vi "BonOMM-SAOMM.Test.vi"() -> ()   [LabVIEW 2011] (continued)
            stop <- w2768 stop-if-true
            # "Commandes Externes sur le PORT SÉRIE et TCP/IP"
            n5059 = local read "CmdFIFO"() -> (w2769:T14)
            n5060 = Array Size(array=w2769) -> (size(s)=w2771:i32)
            n5061 = Greater Than 0?(x=w2771) -> (x > 0?=w2770:bool)
            n5062 = case shown="True" w2770 {
              tunnel: w2769 -> [_ w2779]
              frame False {
                n5063 = local write "ActiveCmd"(T15 {"CmdAct"="", "CmdArgs"="", "Source"=""} ("ActiveCmd")) -> ()
                "CmdPending" <- FALSE
              }
              frame True {
                w2775 = u32 0 ("Output Code")
                # "Enlève les erreurs ..."
                # "Enlève l'élément du FIFO"
                n5064 = stacked-sequence {
                  tunnel: w2779 -> [_ w2793 _]
                  tunnel: [_ w2788 _] -> w2778
                  tunnel: [_ w2787 _] -> w2777
                  tunnel: [_ w2786 _] -> w2776
                  frame #0 {
                    n5065 = control-ref of="FIFO actif"() -> (w2780:refnum<vi>)
                    n5066 = call "Fifo-Wait4Flag.vi"("Raise Flag ?"=TRUE, "Ctl Refnum IN"=w2780) -> ()  [unwired: 8 in, 2 out]
                  }
                  frame #1 {
                    n5067 = local read "CmdDone"() -> (w2784:T14)
                    n5068 = Delete From Array(array=w2793, length=1, index=0) -> (deleted portion=w2789:T14, array with subset deleted=w2790:T14)
                    n5069 = local write "CmdFIFO"(w2790) -> ()
                    n5070 = Index Array(array=w2789) -> (element=w2785:T15)  [unwired: 1 in]
                    "ActiveCmd" <- w2785
                    n5071 = call "PCE-Archive.vi"("Nouvelle Commande"=w2785, "MaxLength"=3, "CmdDone IN"=w2784) -> ("CmdDone OUT"=w2783:T14)  [unwired: 8 in]
                    n5072 = Unbundle By Name(w2785) -> ("CmdAct"=w2788:string, "CmdArgs"=w2787:string, "Source"=w2786:string)
                    n5073 = local write "CmdDone"(w2783) -> ()
                  }
                  frame #2 {
                    n5074 = local write "FIFO actif"(FALSE) -> ()
                  }
                }
                n5075 = stacked-sequence {
                  tunnel: w2778 -> [w2797 _]
                  tunnel: w2777 -> [w2796 _]
                  tunnel: w2776 -> [w2795 w3138]
                  frame #0 {
                    # "Effectue la commande ..."
                    n5076 = case shown="\"EFOY \"" w2797 {
                      tunnel: w2796 -> [_ w2803 w2899 w2907 w2945 w3049 w3057 _]
                      tunnel: w2795 -> [_ _ _ _ _ _ _ _]
                      frame Default {
                        n5077 = local write "ANSW"("Commande non reconnue" ("ANSW")) -> ()
                      }
                      frame "ETCS" {
                        # "Commandes vers TCS"
                        n5078 = call "ETCS_decodeur.vi"("chaine entree"=w2803) -> ("Args"=w2800:dbl[], "nb args"=w2804:i32)  [unwired: 1 out]
                        n5079 = Delete From Array(array=w2800, index=0 ("indice")) -> (deleted portion=w2801:dbl, array with subset deleted=w2799:dbl[])  [unwired: 1 in]
                        n5080 = To Long Integer(number=w2801) -> (32bit integer=w2805:i32)
                        n5081 = case shown="27" w2805 {
                          selector: w2805 -> [_ w2816 _ w2881]
                          tunnel: w2804 -> [_ w2817 w2851 _]
                          tunnel: w2799 -> [_ w2815 _ w2880]
                          frame 0, Default {
                            w2806 = u32 128 ("Bit to add")
                            n5082 = local read "Warning Code"() -> (w2810:u32)
                            n5083 = local read "FIFO d'erreur"() -> (w2808:T7)
                            n5084 = local read "Error Code"() -> (w2809:u32)
                            n5085 = call "Error_Format.vi"("FIFO IN"=w2808, "Error Code IN"=w2809, "Warning Code IN"=w2810, "Error Bit"=w2806, "Warning Bit"=w2806, "Source"="ETCS", "Comment"="Commande non-supportée/indéfinie") -> ("FIFO OUT"=w2811:T7, "Error Code OUT"=w2812:u32, "Warning Code OUT"=w2813:u32)  [unwired: 10 in]
                            n5086 = local write "Warning Code"(w2813) -> ()
                            n5087 = local write "FIFO d'erreur"(w2811) -> ()
                            n5088 = local write "Error Code"(w2812) -> ()
                          }
                          frame 6, 14..16, 22 {
                            # "Vérifie le nombre d'arguments ..."
                            # "Envoir des commandes sans gestions ni réponse de TCS"
                            n5089 = case shown="6" w2816 {
                              tunnel: w2817 -> [w2843 w2844 w2849]
                              tunnel: [w2841 w2845 w2847] -> w2818
                              frame Default {
                                n5090 = Equal?(x=w2843, y=1) -> (x = y?=w2841:bool)
                              }
                              frame 6 {
                                n5091 = Equal?(x=w2844, y=3) -> (x = y?=w2845:bool)
                              }
                              frame 14 {
                                n5092 = Equal?(x=w2849, y=4) -> (x = y?=w2847:bool)
                              }
                            }
                            n5093 = case shown="True" w2818 {
                              tunnel: w2815 -> [_ w2826]
                              tunnel: w2816 -> [_ w2825]
                              frame False {
                                # "Nombre d'arguments incorrect"
                                n5094 = local read "Error Code"() -> (w2821:u32)
                                n5095 = Or(x=w2821, y=u32 128) -> (x .or. y?=w2820:u32)
                                n5096 = local write "Error Code"(w2820) -> ()
                              }
                              frame True {
                                n5097 = local read "TCS VRN"() -> (w2824:refnum<visa-resource-name>)
                                n5098 = control-ref of="TCS actif"() -> (w2822:refnum<vi>)
                                n5099 = call "EXCOM-CMD.vi"("VRN IN"=w2824, "Bool Refnum"=w2822, "Commande #"=w2825, "Args"=w2826) -> ("VRN OUT"=w2823:refnum<visa-resource-name>, "Error OUT"=w2827:errorcluster)  [unwired: 9 in, 1 out]
                                n5100 = local write "TCS VRN"(w2823) -> ()
                                n5101 = case shown="Error" w2827 {
                                tunnel: w2825 -> [_ w2838]
                                frame No Error {
                                }
                                frame Error {
                                w2828 = u32 4
                                n5102 = local read "Warning Code"() -> (w2834:u32)
                                n5103 = local read "FIFO d'erreur"() -> (w2836:T7)
                                n5104 = local read "Error Code"() -> (w2835:u32)
                                n5105 = Number To Decimal String(number=w2838) -> (decimal integer string=w2837:string)  [unwired: 1 in]
                                n5106 = Concatenate Strings("Erreur lors de l'envoie de la commande #", w2837, ", vérifiez la communication sur le port TCS C ...") -> (w2833:string)
                                n5107 = call "Error_Format.vi"("FIFO IN"=w2836, "Error Code IN"=w2835, "Warning Code IN"=w2834, "Error Bit"=w2828, "Warning Bit"=w2828, "Source"="ETCS", "Comment"=w2833) -> ("FIFO OUT"=w2832:T7, "Error Code OUT"=w2831:u32, "Warning Code OUT"=w2830:u32)  [unwired: 10 in]
                                n5108 = local write "Warning Code"(w2830) -> ()
                                n5109 = local write "FIFO d'erreur"(w2832) -> ()
                                n5110 = local write "Error Code"(w2831) -> ()
                                }
                                }
                              }
                            }
                          }
                          frame 4 {
                            # "Commande de rotation semie-automatisée ..."
                            n5111 = Equal?(x=w2851, y=2) -> (x = y?=w2852:bool)
                            n5112 = case shown="True" w2852 {
                              frame False {
                                n5113 = local read "Warning Code"() -> (w2859:u32)
                                n5114 = local read "FIFO d'erreur"() -> (w2861:T7)
                                n5115 = local read "Error Code"() -> (w2860:u32)
                                n5116 = call "Error_Format.vi"("FIFO IN"=w2861, "Error Code IN"=w2860, "Warning Code IN"=w2859, "Warning Bit"=u32 128, "Source"="ETCS", "Comment"="Nombre d'arguments incompatibles") -> ("FIFO OUT"=w2857:T7, "Error Code OUT"=w2856:u32, "Warning Code OUT"=w2855:u32)  [unwired: 11 in]
                                n5117 = local write "Warning Code"(w2855) -> ()
                                n5118 = local write "FIFO d'erreur"(w2857) -> ()
                                n5119 = local write "Error Code"(w2856) -> ()
                              }
                              frame True {
                                n5120 = flat-sequence {
                                tunnel: [w2864] -> w2862
                                tunnel: w2862 -> [w2870]
                                frame #0 {
                                w2863 = TRUE ("Value (Signaling)")
                                n5121 = local write "CmdPending"(w2863) -> ()
                                n5122 = property on="ModifRotation" class="Bool (strict)"("Val(Sgnl)"=w2863) -> ()  [unwired: 2 in, 2 out]
                                }
                                frame #1 {
                                n5123 = while {
                                tunnel: [w2865] -> w2864
                                i -> [w2869]
                                stop <- w2868 stop-if-true
                                # "Time-out de 5 minutes ..."
                                n5124 = local read "CmdPending"() -> (w2865:bool)
                                n5125 = Wait (ms)(milliseconds to wait=u32 100) -> ()  [unwired: 1 out]
                                n5126 = call "Max-iteration.vi"("i max"=3000, "i act"=w2869, "Valeur entrante"=w2865) -> ("break ?"=w2868:bool)
                                }
                                }
                                frame #2 {
                                n5127 = case shown="True" w2870 {
                                frame False {
                                }
                                frame True {
                                n5128 = local read "Warning Code"() -> (w2875:u32)
                                n5129 = local read "FIFO d'erreur"() -> (w2877:T7)
                                n5130 = local read "Error Code"() -> (w2876:u32)
                                n5131 = call "Error_Format.vi"("FIFO IN"=w2877, "Error Code IN"=w2876, "Warning Code IN"=w2875, "Warning Bit"=u32 64 ("Bit to add"), "Source"="ETCS", "Comment"="Délai alloué à la commande dépassé !!!") -> ("FIFO OUT"=w2874:T7, "Error Code OUT"=w2873:u32, "Warning Code OUT"=w2872:u32)  [unwired: 11 in]
                                n5132 = local write "Warning Code"(w2872) -> ()
                                n5133 = local write "FIFO d'erreur"(w2874) -> ()
                                n5134 = local write "Error Code"(w2873) -> ()
                                }
                                }
                                }
                                }
                              }
                            }
                          }
                          frame 27 {
                            n5135 = local read "TCS VRN"() -> (w2883:refnum<visa-resource-name>)
                            n5136 = control-ref of="TCS actif"() -> (w2885:refnum<vi>)
                            n5137 = call "EXCOM-CMD.vi"("VRN IN"=w2883, "Bool Refnum"=w2885, "Commande #"=w2881, "Args"=w2880) -> ("VRN OUT"=w2884:refnum<visa-resource-name>, "Error OUT"=w2882:errorcluster)  [unwired: 9 in, 1 out]
                            n5138 = local write "TCS VRN"(w2884) -> ()
                            n5139 = case shown="Error" w2882 {
                              tunnel: w2881 -> [_ w2896]
                              frame No Error {
                              }
                              frame Error {
                                w2886 = u32 4
                                n5140 = local read "Warning Code"() -> (w2892:u32)
                                n5141 = local read "FIFO d'erreur"() -> (w2894:T7)
                                n5142 = local read "Error Code"() -> (w2893:u32)
                                n5143 = Number To Decimal String(number=w2896) -> (decimal integer string=w2895:string)  [unwired: 1 in]
                                n5144 = Concatenate Strings("Erreur lors de l'envoie de la commande #", w2895, ", vérifiez la communication sur le port TCS C ...") -> (w2891:string)
                                n5145 = call "Error_Format.vi"("FIFO IN"=w2894, "Error Code IN"=w2893, "Warning Code IN"=w2892, "Error Bit"=w2886, "Warning Bit"=w2886, "Source"="ETCS", "Comment"=w2891) -> ("FIFO OUT"=w2890:T7, "Error Code OUT"=w2889:u32, "Warning Code OUT"=w2888:u32)  [unwired: 10 in]
                                n5146 = local write "Warning Code"(w2888) -> ()
                                n5147 = local write "FIFO d'erreur"(w2890) -> ()
                                n5148 = local write "Error Code"(w2889) -> ()
                              }
                            }
                          }
                        }
                      }
                      frame "ETAB" {
                        n5149 = call "ETAB_decodeur.vi"("chaine entree"=w2899) -> ("Args"=w2900:string[], "OK done"=w2901:bool)  [unwired: 1 out]
                        n5150 = case shown="False" w2901 {
                          tunnel: w2900 -> [_ w2903]
                          frame False {
                          }
                          frame True {
                            n5151 = Delete From Array(array=w2903, index=0 ("indice")) -> (deleted portion=w2904:string, array with subset deleted=w2902:string[])  [unwired: 1 in]
                            n5152 = case shown="\"STOP\"" w2904 {
                              tunnel: w2902 -> [_ _ _]
                              frame "", Default {
                              }
                              frame "MOVE" {
                              }
                              frame "STOP" {
                              }
                            }
                          }
                        }
                      }
                      frame "EINF" {
                        n5153 = Decimal String To Number(string=w2907) -> (number=w2908:i32)  [unwired: 2 in, 1 out]
                        n5154 = case shown="0, Default" w2908 {
                          tunnel: [w2912 w2932 "" w2940] -> w2906
                          frame 0, Default {
                            w2913 = "\n"
                            n5155 = Get Date/Time In Seconds() -> (seconds since 1Jan1904=w2911:timestamp)
                            n5156 = local read "Q String"() -> (w2914:string)
                            n5157 = To Double Precision Float(number=w2911) -> (double precision float=w2917:dbl)
                            n5158 = Get Date/Time String(seconds (now)=w2917, want seconds? (F)=TRUE) -> (date string=w2916:string, time string=w2915:string)  [unwired: 1 in]
                            n5159 = Concatenate Strings(w2916, w2913, w2915, w2913, w2914, w2913, "") -> (w2912:string)
                          }
                          frame 1 {
                            w2934 = "Ferme ta yeule, va t'en chez vous! -> "
                            n5160 = local read "Q String"() -> (w2926:string)
                            n5161 = Random Number (0-1)() -> (number: 0 to 1=w2929:dbl)
                            n5162 = Number To Fractional String(number=w2929, precision (6)=i16 12) -> (F-format string=w2927:string)  [unwired: 2 in]
                            n5163 = String Length(string=w2934) -> (length=w2937:i32)
                            n5164 = Number To Decimal String(number=w2937, width (-)=i16 8) -> (decimal integer string=w2935:string)
                            n5165 = Search and Replace String(replace all?=TRUE ("replace all? (F)"), input string=w2926, search string=",", replace string="\r" ("replace string (\"\")")) -> (result string=w2919:string)  [unwired: 4 in, 3 out]
                            n5166 = Concatenate Strings("ANSW", w2935, w2934, w2927) -> (w2931:string)
                            n5167 = Search and Replace String(replace all?=TRUE ("replace all? (F)"), input string=w2919, search string=";", replace string="\r" ("replace string (\"\")")) -> (result string=w2918:string)  [unwired: 4 in, 3 out]
                            n5168 = Select(t=w2918, s=TRUE, f=w2931) -> (s? t:f=w2932:string)
                          }
                          frame 2 {
                          }
                          frame 3 {
                            n5169 = Get Date/Time In Seconds() -> (seconds since 1Jan1904=w2939:timestamp)
                            n5170 = To Double Precision Float(number=w2939) -> (double precision float=w2944:dbl)
                            n5171 = Get Date/Time String(seconds (now)=w2944) -> (date string=w2943:string, time string=w2942:string)  [unwired: 2 in]
                            n5172 = Concatenate Strings(w2943, "\n", w2942) -> (w2940:string)
                          }
                        }
                        n5173 = local write "ANSW"(w2906) -> ()
                      }
                      frame "EOFF" {
                        n5174 = call "ETAB_decodeur.vi"("chaine entree"=w2945) -> ("Args"=w2946:string[], "nb args"=w2948:u16)  [unwired: 1 out]
                        n5175 = Equal?(x=w2948, y=u16 3) -> (x = y?=w2947:bool)
                        n5176 = case shown="True" w2947 {
                          tunnel: w2946 -> [_ w2959]
                          frame False {
                          }
                          frame True {
                            # "Warning Code"
                            # "Error Code"
                            # "Causait erreur\ncode CYGA à modifier"
                            n5177 = Index Array(array=w2959, index #1=0 ("indice"), index #2=1 ("indice"), index #3=2 ("indice")) -> (element #1=w2950:string, element #2=w2953:string, element #3=w2954:string)
                            n5178 = Fract/Exp String To Number(string=w2954) -> (number=w2951:dbl)  [unwired: 3 in, 1 out]
                            n5179 = Fract/Exp String To Number(string=w2953) -> (number=w2952:dbl)  [unwired: 3 in, 1 out]
                            n5180 = stacked-sequence {
                              seq-local: [_ w2977 _] -> [_ _ w3020]
                              seq-local: [_ w3002 _] -> [_ _ w3016]
                              seq-local: [_ w3001 _] -> [_ _ w3017]
                              tunnel: w2951 -> [w2969 w2983 _]
                              tunnel: w2952 -> [w2968 w2984 _]
                              frame #0 {
                                n5181 = local write "Offset RA"(w2968) -> ()
                                n5182 = local write "Offset DEC"(w2969) -> ()
                                n5183 = Number To Fractional String(number=w2968, precision (6)=i16 2) -> (F-format string=w2963:string)  [unwired: 2 in]
                                n5184 = Number To Fractional String(number=w2969, precision (6)=i16 2) -> (F-format string=w2962:string)  [unwired: 2 in]
                                n5185 = control-ref of="TERMINAL"() -> (w2971:refnum<vi>)
                                n5186 = control-ref of="Indicateur d'état"() -> (w2970:refnum<vi>)
                                n5187 = Concatenate Strings("Envoi externe d'un offset de " ("string"), w2963, ", " ("string"), w2962) -> (w2961:string)
                                n5188 = call "TERMINAL.vi"("Indicateur Refnum"=w2970, "Terminal Refnum"=w2971, "Indicateur d'état"=w2961) -> ()
                                n5189 = local write "Offset en cours"(TRUE ("enfoncé")) -> ()
                              }
                              frame #1 {
                                w3004 = u32 0 ("Error Code IN")
                                n5190 = control-ref of="MovingXY"() -> (w2973:refnum<vi>)
                                n5191 = local read "Table VRN"() -> (w2995:refnum<visa-resource-name>)
                                n5192 = control-ref of="Position Z"() -> (w2991:refnum<vi>)
                                n5193 = control-ref of="DiffX"() -> (w2986:refnum<vi>)
                                n5194 = control-ref of="DiffY"() -> (w2987:refnum<vi>)
                                n5195 = control-ref of="SNR"() -> (w2974:refnum<vi>)
                                n5196 = local read "TCS VRN"() -> (w2997:refnum<visa-resource-name>)
                                n5197 = local read "Table Error"() -> (w2994:errorcluster)
                                n5198 = control-ref of="TCS actif"() -> (w2993:refnum<vi>)
                                n5199 = control-ref of="Table actif"() -> (w2992:refnum<vi>)
                                n5200 = control-ref of="StartServo"() -> (w2990:refnum<vi>)
                                n5201 = control-ref of="Mode"() -> (w2985:refnum<vi>)
                                n5202 = control-ref of="Servo"() -> (w2989:refnum<vi>)
                                n5203 = control-ref of="StopServo"() -> (w2988:refnum<vi>)
                                n5204 = local read "TCS Error"() -> (w2996:errorcluster)
                                n5205 = local read "TableAstrom"() -> (w2998:T4)
                                n5206 = local read "FieldAstrom"() -> (w3000:T4)
                                n5207 = local read "GuiderAstrom"() -> (w2999:T4)
                                n5208 = Bundle("TCS VRN"=w2997, "TCS Error"=w2996, "Table VRN"=w2995, "Table Error"=w2994) -> (w2982:T41)  [unwired: 1 in]
                                n5209 = Bundle("TableAstrom"=w2998, "FieldAstrom"=w3000, "GuiderAstrom"=w2999) -> (w2981:T40)  [unwired: 1 in]
                                n5210 = Bundle("TCS actif"=w2993, "Table actif"=w2992, "Position Z"=w2991, "StartServo"=w2990, "Mode"=w2985, "Servo"=w2989, "StopServo"=w2988, "DiffX"=w2986, "DiffY"=w2987, "SNR"=w2974, "MovingXY"=w2973) -> (w2980:T42)  [unwired: 1 in]
                                n5211 = call "Cheesy_Offset.vi"("Communications_Cluster"=w2982, "Astrom_Cluster"=w2981, "RA offset"=w2984, "DEC offset"=w2983, "VariablesReferences"=w2980, "OffsetAccuracy (pixels)"="OffsetAcc") -> ("Error code"=w2979:u8, "Undo offset"=w2977:bool, "Warning code"=w2978:u8, "Error Comment"=w2975:string)  [unwired: 6 in]
                                n5212 = while {
                                tunnel: [FALSE] -> w2972
                                stop <- w3011 continue-if-true
                                n5213 = local read "enfoncé"() -> (w3013:bool)
                                n5214 = Not(x=w3013) -> (.not. x?=w3012:bool)
                                n5215 = Wait (ms)(milliseconds to wait=u32 200) -> ()  [unwired: 1 out]
                                n5216 = local write "enfoncé"(w3012) -> ()
                                n5217 = local read "Offset en cours"() -> (w3011:bool)
                                }
                                n5218 = To Unsigned Long Integer(number=w2979) -> (unsigned 32bit integer=w3001:u32)
                                n5219 = To Unsigned Long Integer(number=w2978) -> (unsigned 32bit integer=w3002:u32)
                                n5220 = local read "FIFO d'erreur"() -> (w3005:T7)
                                n5221 = call "Error_Format.vi"("FIFO IN"=w3005, "Error Code IN"=w3004, "Warning Code IN"=w3004, "Error Bit"=w3001, "Warning Bit"=w3002, "Source"="offset", "Comment"=w2975) -> ("FIFO OUT"=w3006:T7)  [unwired: 10 in, 2 out]
                                n5222 = flat-sequence {
                                tunnel: w3006 -> [w3007]
                                frame #0 {
                                n5223 = local write "FIFO d'erreur"(w3007) -> ()
                                }
                                frame #1 {
                                n5224 = local write "Offset en cours"(FALSE) -> ()
                                }
                                }
                                n5225 = local write "enfoncé"(w2972) -> ()
                              }
                              frame #2 {
                                w3022 = FALSE
                                w3015 = FALSE
                                # "Préparation de la réponse ..."
                                n5226 = local write "Offset OK"(w3015) -> ()
                                n5227 = local write "TCS actif"(w3015) -> ()
                                n5228 = local write "RangeTable"(w3022) -> ()
                                n5229 = local write "Calibration"(w3022) -> ()
                                n5230 = local write "stoptable"(w3022) -> ()
                                n5231 = local write "Alacible"(w3022) -> ()
                                n5232 = local write "Origine"(w3022) -> ()
                                n5233 = local write "Centre"(w3022) -> ()
                                n5234 = local read "TERMINAL"() -> (w3026:string)
                                n5235 = Greater Than 0?(x=w3017) -> (x > 0?=w3018:bool)
                                n5236 = case shown="True" w3018 {
                                tunnel: [w3029 w3033] -> w3019
                                tunnel: w3017 -> [_ w3032]
                                tunnel: w3016 -> [w3028 _]
                                frame False {
                                n5237 = Number To Decimal String(number=w3028) -> (decimal integer string=w3031:string)  [unwired: 1 in]
                                n5238 = Concatenate Strings("W" ("string"), w3031) -> (w3029:string)
                                }
                                frame True {
                                n5239 = Number To Decimal String(number=w3032) -> (decimal integer string=w3035:string)  [unwired: 1 in]
                                n5240 = Concatenate Strings("E" ("string"), w3035) -> (w3033:string)
                                }
                                }
                                n5241 = Select(t=" : échoué" ("Command String"), s=w3020, f=" : réussi" ("Command String")) -> (s? t:f=w3027:string)
                                n5242 = Concatenate Strings(w3026, w3027) -> (w3025:string)
                                n5243 = local write "TERMINAL"(w3025) -> ()
                                n5244 = Select(t=w3019, s=w3020, f="OK" ("Command String")) -> (s? t:f=w3014:string)
                                n5245 = local write "ANSW"(w3014) -> ()
                                n5246 = case shown="True" w3020 {
                                frame False {
                                }
                                frame True {
                                n5247 = local read "Table VRN"() -> (w3040:refnum<visa-resource-name>)
                                n5248 = control-ref of="Table actif"() -> (w3038:refnum<vi>)
                                n5249 = local read "Table Error"() -> (w3037:errorcluster)
                                n5250 = control-ref of="TCS actif"() -> (w3041:refnum<vi>)
                                n5251 = local read "TCS VRN"() -> (w3042:refnum<visa-resource-name>)
                                n5252 = call "EXCOM-CMD.vi"("VRN IN"=w3042, "Bool Refnum"=w3041, "Commande #"=13) -> ("VRN OUT"=w3043:refnum<visa-resource-name>, "Error OUT"=w3044:errorcluster)  [unwired: 10 in, 1 out]
                                n5253 = call "Newmark-Stop.vi"("Table VRN IN"=w3040, "Bool Refnum"=w3038, "Error IN"=w3037) -> ("Table VRN OUT"=w3039:refnum<visa-resource-name>, "Error OUT"=w3036:errorcluster)  [unwired: 11 in]
                                n5254 = local write "Table Error"(w3036) -> ()
                                n5255 = local write "Table VRN"(w3039) -> ()
                                n5256 = local write "TCS VRN"(w3043) -> ()
                                n5257 = local write "TCS Error"(w3044) -> ()
                                }
                                }
                              }
                            }
                            n5258 = Not Equal?(x=w2950, y="N") -> ()  [unwired: 1 out]
                          }
                        }
                      }
                      frame "EFOY " {
                        # "Permet d'effectuer des ajustements au foyer"
                        n5259 = local read "Foyer"() -> (w3046:dbl)
                        n5260 = Fract/Exp String To Number(string=w3049, default (0 dbl)=w3046) -> (number=w3048:dbl)  [unwired: 2 in, 1 out]
                        n5261 = Not Equal To 0?(x=w3048) -> (x != 0?=w3047:bool)
                        n5262 = case shown="True" w3047 {
                          tunnel: w3048 -> [_ w3052]
                          tunnel: w3046 -> [_ w3051]
                          frame False {
                          }
                          frame True {
                            n5263 = Bundle By Name(cluster=T22 {"newFoyer"=0.0, "updSonde"=TRUE, "oldFoyer"=0.0}, "newFoyer"=w3052, "updSonde"=TRUE, "oldFoyer"=w3051) -> (w3053:T22)
                            n5264 = call "EnqueueEvents.vi"("data"=w3053, "message"="Foyer.Ajuster") -> ()  [unwired: 1 in]
                          }
                        }
                      }
                      frame "ERAF" {
                        n5265 = call "ETAB_decodeur.vi"("chaine entree"=w3057) -> ("Args"=w3060:string[])  [unwired: 2 out]
                        n5266 = Index Array(array=w3060) -> (element=w3059:string)  [unwired: 1 in]
                        n5267 = local read "MC-BonOMM VRN"() -> (w3058:refnum<visa-resource-name>)
                        n5268 = local read "Excmd VRN"() -> (w3056:refnum<visa-resource-name>)
                        n5269 = case shown="\"1\", \"2\", \"3\", \"4\", \"5\", \"6\"" w3059 {
                          selector: w3059 -> [_ _ _ w3099 _]
                          tunnel: w3058 -> [_ w3066 w3082 _ _]
                          tunnel: w3056 -> [_ w3061 w3077 w3096 w3125]
                          frame "", Default {
                          }
                          frame "m" {
                            n5270 = call "MC-BonOMM_talker.vi"("MC-BonOMM VRN"=w3066, "Commande"="m", "byte count"=u32 1, "answer=command?"=FALSE) -> ("Answer"=w3063:string, "ok ?"=w3062:bool)  [unwired: 1 in]
                            n5271 = case shown="True" w3062 {
                              tunnel: w3063 -> [_ w3069]
                              tunnel: w3061 -> [_ w3074]
                              frame False {
                              }
                              frame True {
                                n5272 = Concatenate Strings(w3069, "\n" ("string")) -> (w3068:string)
                                n5273 = String Length(string=w3068) -> (length=w3076:i32)
                                n5274 = Number To Decimal String(number=w3076, width (-)=i16 4 ("largeur (-)")) -> (decimal integer string=w3072:string)
                                n5275 = Concatenate Strings("ANSW", w3072, w3068) -> (w3071:string)
                                n5276 = VISA Write(VISA resource name=w3074, write buffer=w3071) -> ()  [unwired: 1 in, 3 out]
                              }
                            }
                          }
                          frame "q" {
                            n5277 = call "MC-BonOMM_talker.vi"("MC-BonOMM VRN"=w3082, "Commande"="q", "byte count"=u32 1, "answer=command?"=FALSE) -> ("Answer"=w3079:string, "ok ?"=w3078:bool)  [unwired: 1 in]
                            n5278 = case shown="True" w3078 {
                              tunnel: w3079 -> [_ w3086]
                              tunnel: w3077 -> [_ w3090]
                              frame False {
                              }
                              frame True {
                                n5279 = Concatenate Strings(w3086, "\n" ("string")) -> (w3084:string)
                                n5280 = String Length(string=w3084) -> (length=w3092:i32)
                                n5281 = Number To Decimal String(number=w3092, width (-)=i16 4 ("largeur (-)")) -> (decimal integer string=w3088:string)
                                n5282 = Concatenate Strings("ANSW", w3088, w3084) -> (w3087:string)
                                n5283 = VISA Write(VISA resource name=w3090, write buffer=w3087) -> ()  [unwired: 1 in, 3 out]
                              }
                            }
                          }
                          frame "1", "2", "3", "4", "5", "6" {
                            n5284 = Decimal String To Number(string=w3099) -> (number=w3100:i32)  [unwired: 2 in, 1 out]
                            n5285 = case shown="6" w3100 {
                              frame 0, Default {
                              }
                              frame 1 {
                                n5286 = property on="filtre #1" class="Bool (strict)"("Value (Signaling)"=TRUE) -> ()  [unwired: 2 in, 2 out]
                              }
                              frame 2 {
                                n5287 = property on="filtre #2" class="Bool (strict)"("Value (Signaling)"=TRUE) -> ()  [unwired: 2 in, 2 out]
                              }
                              frame 3 {
                                n5288 = property on="filtre #3" class="Bool (strict)"("Value (Signaling)"=TRUE) -> ()  [unwired: 2 in, 2 out]
                              }
                              frame 4 {
                                n5289 = property on="filtre #4" class="Bool (strict)"("Value (Signaling)"=TRUE) -> ()  [unwired: 2 in, 2 out]
                              }
                              frame 5 {
                                n5290 = property on="filtre #5" class="Bool (strict)"("Value (Signaling)"=TRUE) -> ()  [unwired: 2 in, 2 out]
                              }
                              frame 6 {
                                n5291 = property on="filtre #6" class="Bool (strict)"("Value (Signaling)"=TRUE) -> ()  [unwired: 2 in, 2 out]
                              }
                            }
                            n5292 = while {
                              tunnel: w3096 -> [_]
                              tunnel: w3100 -> [w3123]
                              tunnel: [FALSE ("Bypass Tech")] -> w3097
                              tunnel: [w3117] -> w3094
                              tunnel: [w3116] -> w3093
                              i -> [w3121]
                              stop <- w3122 stop-if-true
                              n5293 = local read "F#"() -> (w3117:i32)
                              n5294 = Wait (ms)(milliseconds to wait=u32 200) -> ()  [unwired: 1 out]
                              n5295 = Equal?(x=w3117, y=w3123) -> (x = y?=w3116:bool)
                              n5296 = call "Max-iteration.vi"("i max"=150, "i act"=w3121, "Valeur entrante"=w3116) -> ("break ?"=w3122:bool)
                            }
                            n5297 = Number To Decimal String(number=w3094) -> (decimal integer string=w3095:string)  [unwired: 1 in]
                            n5298 = case shown="False" w3093 {
                              tunnel: w3096 -> [_ w3107]
                              tunnel: w3095 -> [_ w3101]
                              frame False {
                              }
                              frame True {
                                n5299 = Concatenate Strings(w3101, "\n" ("string")) -> (w3102:string)
                                n5300 = String Length(string=w3102) -> (length=w3109:i32)
                                n5301 = Number To Decimal String(number=w3109, width (-)=i16 4 ("largeur (-)")) -> (decimal integer string=w3105:string)
                                n5302 = Concatenate Strings("ANSW", w3105, w3102) -> (w3104:string)
                                n5303 = VISA Write(VISA resource name=w3107, write buffer=w3104) -> ()  [unwired: 1 in, 3 out]
                              }
                            }
                            n5304 = local write "Bypass Tech"(w3097) -> ()
                            "Bypass Tech" <- TRUE ("Bypass Tech")
                          }
                          frame "i" {
                            n5305 = local read "Tableau des filtres"() -> (w3132:string[])
                            n5306 = local write "string temporaire"("") -> ()
                            n5307 = for {
                              tunnel: w3132 -> [w3136] mode=indexing
                              tunnel: [w3133] -> w3124
                              n5308 = Concatenate Strings("string temporaire", w3136, "\n" ("string")) -> (w3133:string)
                              n5309 = local write "string temporaire"(w3133) -> ()
                            }
                            n5310 = String Length(string=w3124) -> (length=w3130:i32)
                            n5311 = Number To Decimal String(number=w3130, width (-)=i16 4 ("largeur (-)")) -> (decimal integer string=w3127:string)
                            n5312 = Concatenate Strings("ANSW", w3127, w3124) -> (w3126:string)
                            n5313 = VISA Write(VISA resource name=w3125, write buffer=w3126) -> ()  [unwired: 1 in, 3 out]
                          }
                        }
                      }
                      frame "EHEX" {
                      }
                    }
                  }
                  frame #1 {
                    # "Envoie la réponse sur le port approprié"
                    n5314 = String Subset(string=w3138, length (rest)=3 ("length (rest)")) -> (substring=w3140:string)  [unwired: 1 in]
                    n5315 = Equal?(x=w3140, y="COM") -> (x = y?=w3139:bool)
                    n5316 = case shown="False" w3139 {
                      tunnel: w3138 -> [w3153 w3165]
                      tunnel: "ANSW" -> [w3145 w3157]
                      frame False {
                        # "Réponse TCP/IP"
                        n5317 = Type Cast(type=refnum<k5> refnum ("connection ID out"), x=w3153) -> (*(type *) &x=w3152:refnum<k5>)
                        n5318 = String Length(string=w3145) -> (length=w3149:i32)
                        n5319 = Number To Decimal String(number=w3149, width (-)=i16 8) -> (decimal integer string=w3147:string)
                        n5320 = Concatenate Strings("ANSW", w3147, w3145) -> (w3144:string)
                        n5321 = TCP Write(connection ID=w3152, data in=w3144, 9:500 ("timeout ms (25000)")) -> (error out=w3150:errorcluster)  [unwired: 1 in, 2 out]
                        n5322 = local write "TCP/IP Error"(w3150) -> ()
                      }
                      frame True {
                        # "Réponse sur le port Série ..."
                        n5323 = local read "Excmd VRN"() -> (w3166:refnum<visa-resource-name>)
                        n5324 = Type Cast(type=w3166, x=w3165) -> (*(type *) &x=w3164:refnum<visa-resource-name>)
                        n5325 = Concatenate Strings(w3157, "\n") -> (w3158:string)
                        n5326 = String Length(string=w3158) -> (length=w3162:i32)
                        n5327 = Number To Decimal String(number=w3162, width (-)=i16 4) -> (decimal integer string=w3161:string)
                        n5328 = Concatenate Strings("ANSW", w3161, w3158) -> (w3159:string)
                        n5329 = local read "Excom Error"() -> (w3155:errorcluster)
                        n5330 = VISA Write(VISA resource name=w3164, write buffer=w3159, error in (no error)=w3155) -> (error out=w3154:errorcluster)  [unwired: 2 out]
                        n5331 = local write "Excom Error"(w3154) -> ()
                      }
                    }
                  }
                }
                "Error Code" <- w2775
                "Warning Code" <- w2775
              }
            }
            n5332 = Wait Until Next ms Multiple(millisecond multiple=u32 50 ("n millisecondes")) -> ()  [unwired: 1 out]
            n5333 = local read "Quit"() -> (w2768:bool)
          }
          "Gestion Scripts" <- w944
          n5334 = while {
            tunnel: w957 -> [w1030]
            tunnel: [w1026] -> w947
            stop <- w1026 stop-if-true
            # "ms to wait for 1st 4 bytes"
            n5335 = local read "Signature"() -> (w1035:u32)
            n5336 = local read "PrAMS Error"() -> (w1032:errorcluster)
            n5337 = local read "Hexapod VRN"() -> (w1031:refnum<visa-resource-name>)
            n5338 = local read "MessageType"() -> (w1033:cluster{string[], u32[]})
            n5339 = call "PRAMMS-LISTENER.vi"("PRAMMS-COMM IN"=w1031, "Bool Refnum"=w1030, "MessageTypeArray"=w1033, "Signature"=w1035, "Error IN"=w1032, "ReadTimeOut"=5) -> ("Type"=w1028:string, "ByteArray"=w1027:u8[], "Received?"=w1029:bool)  [unwired: 4 in, 3 out]
            n5340 = case shown="True" w1029 {
              tunnel: w1028 -> [_ w1037]
              tunnel: w1027 -> [_ w1036]
              frame False {
              }
              frame True {
                n5341 = case shown="\"emtAcknowledgment\"" w1037 {
                  selector: w1037 -> [w1039 _ _ w1068 _ _ w1090 _ _ _]
                  tunnel: w1036 -> [w1038 w1055 _ w1067 w1088 _ w1091 _ _ w1142]
                  frame Default {
                    n5342 = Type Cast(x=w1038) -> (*(type *) &x=w1043:string)  [unwired: 1 in]
                    n5343 = local read "Dump"() -> (w1040:string)
                    n5344 = Concatenate Strings(w1040, w1039, " : " ("string"), w1043, "\r") -> (w1044:string)
                    n5345 = local read "nDumped"() -> (w1046:i32)
                    n5346 = Increment(x=w1046) -> (x+1=→"nDumped":i32)
                    n5347 = local write "Dump"(w1044) -> ()
                  }
                  frame "emtError" {
                    # "Rempli le fifo d'erreur"
                    # "Si un code d'erreur est retourné, il sera mis négatif et entrez dans la variable ACK"
                    n5348 = To Unsigned Long Integer(number=u32 0) -> (unsigned 32bit integer=w1053:u32)
                    n5349 = call-poly "SAOMM-EXTRACT-DATA.vi"("UINT32"=w1053, "Data"=w1055) -> ("Value"=w1050:u32)  [unwired: 10 in, 3 out]
                    n5350 = Negate(x=1) -> (-x=w1047:i32)
                    n5351 = Not Equal To 0?(x=w1050) -> (x != 0?=w1051:bool)
                    n5352 = local write "Hexapod-ACK"(w1047) -> ()
                    n5353 = case shown="False" w1051 {
                      tunnel: w1050 -> [_ w1063]
                      tunnel: ["Erreur reçu de l'Hexapode (code : indéfini)" w1059] -> w1049
                      frame False {
                      }
                      frame True {
                        n5354 = Number To Decimal String(number=w1063) -> (decimal integer string=w1062:string)  [unwired: 1 in]
                        n5355 = Concatenate Strings("Erreur reçu de l'Hexapode (code : ", w1062, ")") -> (w1059:string)
                      }
                    }
                    n5356 = local read "FIFO d'erreur"() -> (w1057:T7)
                    n5357 = call "Error_Format.vi"("FIFO IN"=w1057, "Error Code IN"=w1050, "Source"="Hexapod", "Comment"=w1049) -> ("FIFO OUT"=w1056:T7)  [unwired: 13 in, 2 out]
                    n5358 = local write "FIFO d'erreur"(w1056) -> ()
                  }
                  frame "emtAcknowledgment" {
                    n5359 = local read "Nb_ACK (hex)"() -> (w1065:i32)
                    n5360 = Increment(x=w1065) -> (x+1=→"Nb_ACK (hex)":i32)
                    "Hexapod-ACK" <- 1
                  }
                  frame "emtUAxis", "emtVAxis", "emtWAxis", "emtXAxis", "emtYAxis", "emtZAxis" {
                    n5361 = To Double Precision Float(number=0.0) -> (double precision float=w1070:dbl)
                    n5362 = call-poly "SAOMM-EXTRACT-DATA.vi"("DBL"=w1070, "Data"=w1067) -> ("Value"=w1071:dbl)  [unwired: 10 in, 3 out]
                    n5363 = case shown="\"emtWAxis\"" w1068 {
                      selector: w1068 -> [w1073 _ _ _ _ _ _]
                      tunnel: w1071 -> [w1076 w1079 w1080 w1081 w1082 w1083 w1084]
                      frame Default {
                        w1075 = "\r"
                        n5364 = Type Cast(type=w1075, x=w1076) -> (*(type *) &x=w1077:string)
                        n5365 = local read "Dump"() -> (w1072:string)
                        n5366 = Concatenate Strings(w1072, w1073, " : " ("string"), w1077, w1075) -> (w1078:string)
                        n5367 = local write "Dump"(w1078) -> ()
                      }
                      frame "emtXAxis" {
                        n5368 = local write "HexX"(w1079) -> ()
                      }
                      frame "emtYAxis" {
                        n5369 = local write "HexY"(w1080) -> ()
                      }
                      frame "emtZAxis" {
                        n5370 = local write "HexZ"(w1081) -> ()
                      }
                      frame "emtUAxis" {
                        n5371 = local write "HexU"(w1082) -> ()
                      }
                      frame "emtVAxis" {
                        n5372 = local write "HexV"(w1083) -> ()
                      }
                      frame "emtWAxis" {
                        n5373 = local write "HexW"(w1084) -> ()
                      }
                    }
                  }
                  frame "emtVelocity" {
                    n5374 = To Double Precision Float(number=0.0) -> (double precision float=w1086:dbl)
                    n5375 = call-poly "SAOMM-EXTRACT-DATA.vi"("DBL"=w1086, "Data"=w1088) -> ("Value"=w1085:dbl)  [unwired: 10 in, 3 out]
                    n5376 = local write "Vitesse [mm/s]"(w1085) -> ()
                  }
                  frame "emtMoveIncrement" {
                    # "Quel format cela aura-t-il"
                  }
                  frame "emtUAxisOffset", "emtVAxisOffset", "emtWAxisOffset", "emtXAxisOffset", "emtYAxisOffset", "emtZAxisOffset" {
                    n5377 = To Double Precision Float(number=0.0) -> (double precision float=w1093:dbl)
                    n5378 = call-poly "SAOMM-EXTRACT-DATA.vi"("DBL"=w1093, "Data"=w1091) -> ("Value"=w1089:dbl)  [unwired: 10 in, 3 out]
                    n5379 = case shown="\"emtWAxisOffset\"" w1090 {
                      selector: w1090 -> [w1095 _ _ _ _ _ _]
                      tunnel: w1089 -> [w1094 w1101 w1102 w1103 w1104 w1105 w1106]
                      frame Default {
                        w1098 = "\r"
                        n5380 = Type Cast(type=w1098, x=w1094) -> (*(type *) &x=w1099:string)
                        n5381 = local read "Dump"() -> (w1096:string)
                        n5382 = Concatenate Strings(w1096, w1095, " : " ("string"), w1099, w1098) -> (w1100:string)
                        n5383 = local write "Dump"(w1100) -> ()
                      }
                      frame "emtXAxisOffset" {
                        n5384 = local write "Offset X"(w1101) -> ()
                      }
                      frame "emtYAxisOffset" {
                        n5385 = local write "Offset Y"(w1102) -> ()
                      }
                      frame "emtZAxisOffset" {
                        n5386 = local write "Offset Z"(w1103) -> ()
                      }
                      frame "emtUAxisOffset" {
                        n5387 = local write "Offset U"(w1104) -> ()
                      }
                      frame "emtVAxisOffset" {
                        n5388 = local write "Offset V"(w1105) -> ()
                      }
                      frame "emtWAxisOffset" {
                        n5389 = flat-sequence {
                          tunnel: w1106 -> [w1107]
                          frame #0 {
                            n5390 = local write "Offset W"(w1107) -> ()
                          }
                          frame #1 {
                            n5391 = local read "HexapodQuery"() -> (w1109:u32)
                            n5392 = Tick Count (ms)() -> (millisecond timer value=w1110:u32)
                            n5393 = local write "QueryingHexapod"(FALSE ("QueryingHexapod")) -> ()
                            n5394 = Subtract(x=w1110, y=w1109) -> (x-y=w1108:u32)
                            n5395 = local write "HexapodQuery"(w1108) -> ()
                          }
                        }
                      }
                    }
                  }
                  frame "emtMoveStarted" {
                    n5396 = local write "HxMoving"(TRUE) -> ()
                  }
                  frame "emtMoveStopped" {
                    n5397 = local write "HxMoving"(FALSE) -> ()
                  }
                  frame "emtMoving" {
                    w1123 = 0.0
                    w1124 = u8[] []
                    # "emtMoving\n\nTimeStamp(U64)\nXAxis(DBL)\nYAxis(DBL)\nZAxis(DBL)\nUAxis(DBL)\nZAxis(DBL)"
                    n5398 = Type Cast(type=dbl[] [], x=w1142) -> (*(type *) &x=w1140:dbl[])
                    n5399 = Index Array(array=w1140) -> (element #1=w1139:dbl, element #2=w1136:dbl, element #3=w1122:dbl, element #4=w1121:dbl, element #5=w1120:dbl, element #6=w1119:dbl)  [unwired: 6 in]
                    n5400 = To Unsigned Quad Integer(1:u64 0) -> (0:w1138:u64)
                    n5401 = Type Cast(type=w1138, x=w1139) -> (*(type *) &x=→"QueryTimeStamp":u64)
                    n5402 = Type Cast(type=w1124, x=w1121) -> (*(type *) &x=w1130:u8[])
                    n5403 = Type Cast(type=w1124, x=w1120) -> (*(type *) &x=w1127:u8[])
                    n5404 = Type Cast(type=w1124, x=w1119) -> (*(type *) &x=w1126:u8[])
                    n5405 = Type Cast(type=w1124, x=w1136) -> (*(type *) &x=w1135:u8[])
                    n5406 = Type Cast(type=w1124, x=w1122) -> (*(type *) &x=w1131:u8[])
                    n5407 = Reverse 1D Array(array=w1135) -> (reversed array=w1134:u8[])
                    n5408 = Reverse 1D Array(array=w1131) -> (reversed array=w1132:u8[])
                    n5409 = Reverse 1D Array(array=w1130) -> (reversed array=w1129:u8[])
                    n5410 = Reverse 1D Array(array=w1127) -> (reversed array=w1128:u8[])
                    n5411 = Reverse 1D Array(array=w1126) -> (reversed array=w1125:u8[])
                    n5412 = Type Cast(type=w1123, x=w1129) -> (*(type *) &x=w1117:dbl)
                    n5413 = Type Cast(type=w1123, x=w1128) -> (*(type *) &x=w1116:dbl)
                    n5414 = Type Cast(type=w1123, x=w1125) -> (*(type *) &x=w1115:dbl)
                    n5415 = Type Cast(type=w1123, x=w1134) -> (*(type *) &x=w1133:dbl)
                    n5416 = Type Cast(type=w1123, x=w1132) -> (*(type *) &x=w1118:dbl)
                    n5417 = local write "HexX"(w1133) -> ()
                    n5418 = local write "HexY"(w1118) -> ()
                    n5419 = local write "HexZ"(w1117) -> ()
                    n5420 = local write "HexU"(w1116) -> ()
                    n5421 = local write "HexV"(w1115) -> ()
                  }
                }
              }
            }
            n5422 = local read "Quit"() -> (w1026:bool)
          }
          "Hexapod Listener" <- w947
          n5423 = while {
            tunnel: [w3870] -> w955
            stop <- w3870 stop-if-true
            # "Structure de gestion des événements prioritaires"
            n5424 = event shown="[2] \"StopTel\": Value Change" {
              selector: _ -> [_ _ _ _]
              dyn-events: _ -> [_ _ _ _]
              timeout: 250 -> [_ _ _ _]
              event Timeout {
                n5425 = event-data() -> ()  [unwired: 1 in, 1 out]
              }
              event "stoptable": Value Change {
                n5426 = event-data() -> ("NewVal"=w3872:bool)  [unwired: 1 in, 4 out]
                n5427 = case shown="True" w3872 {
                  frame False {
                  }
                  frame True {
                    n5428 = flat-sequence {
                      frame #0 {
                        w3873 = FALSE ("stoptable")
                        n5429 = local read "Table VRN"() -> (w3883:refnum<visa-resource-name>)
                        n5430 = local write "CorrectZ"(w3873) -> ()
                        n5431 = local write "CorrectXY"(w3873) -> ()
                        n5432 = local write "CurvCorrect"(w3873) -> ()
                        n5433 = local write "Focusing"(w3873) -> ()
                        n5434 = local write "stoptable"(w3873) -> ()
                        n5435 = control-ref of="Table actif"() -> (w3878:refnum<vi>)
                        n5436 = call "Newmark-Stop.vi"("Table VRN IN"=w3883, "Bool Refnum"=w3878) -> ("Table VRN OUT"=w3882:refnum<visa-resource-name>, "Error OUT"=w3881:errorcluster)  [unwired: 12 in]
                        n5437 = call "Newmark-Clear.vi"("Table VRN IN"=w3882, "Bool Refnum"=w3878, "Error IN"=w3881) -> ("Table VRN OUT"=w3880:refnum<visa-resource-name>, "Error OUT"=w3879:errorcluster)  [unwired: 11 in]
                        n5438 = control-ref of="TERMINAL"() -> (w3876:refnum<vi>)
                        n5439 = control-ref of="Indicateur d'état"() -> (w3877:refnum<vi>)
                        n5440 = local write "Table VRN"(w3880) -> ()
                        n5441 = local write "Table Error"(w3879) -> ()
                        n5442 = property on="Origine" class="Bool (strict)"("Blinking"=FALSE) -> ()  [unwired: 2 in, 2 out]
                        n5443 = call "TERMINAL.vi"("Indicateur Refnum"=w3877, "Terminal Refnum"=w3876, "Indicateur d'état"="Arrêt d'urgence des tables") -> ()
                      }
                      frame #1 {
                        # "Arrêt de l'initialisation des tables ..."
                        # "Wait for the stages to stop"
                        n5444 = while {
                          i -> [w3892]
                          stop <- w3893 stop-if-true
                          n5445 = local read "MovingXY"() -> (w3889:bool)
                          n5446 = Wait (ms)(milliseconds to wait=u32 250) -> ()  [unwired: 1 out]
                          n5447 = Greater?(x=w3892, y=5) -> (0:w3890:bool)
                          n5448 = Not(x=w3889) -> (.not. x?=w3888:bool)
                          n5449 = Or(x=w3888, y=w3890) -> (x .or. y?=w3893:bool)
                        }
                        n5450 = local read "Origine en cours..."() -> (w3884:bool)
                        n5451 = case shown="True" w3884 {
                          selector: w3884 -> [_ w3885]
                          frame False {
                          }
                          frame True {
                            n5452 = while {
                              stop <- w3887 continue-if-true
                              n5453 = local read "Origine en cours..."() -> (w3887:bool)
                              n5454 = Wait (ms)(milliseconds to wait=u32 50) -> ()  [unwired: 1 out]
                            }
                            "Quit_Origine" <- w3885
                          }
                        }
                      }
                      frame #2 {
                        w3895 = FALSE
                        # "Remise à zéro des exceptions ..."
                        n5455 = flat-sequence {
                          frame #0 {
                            n5456 = control-ref of="Table actif"() -> (w3900:refnum<vi>)
                            n5457 = call "Newmark-Wait4Flag.vi"("Raise Flag ?"=TRUE, "Ctl Refnum IN"=w3900) -> ()  [unwired: 8 in, 2 out]
                          }
                          frame #1 {
                            n5458 = local write "Exceptions"(T3 {"Command Error"=FALSE, "Slip/Stall"=FALSE, "Overtravel"=FALSE, "Done"=FALSE, "nError"=0, "nSlip"=0, "nOT"=0, "nDone"=0} ("Exceptions")) -> ()
                          }
                          frame #2 {
                            n5459 = local write "Table actif"(FALSE ("Table actif")) -> ()
                          }
                        }
                        n5460 = local read "Position X"() -> (w3898:dbl)
                        n5461 = local read "Position Y"() -> (w3897:dbl)
                        n5462 = local read "Position Z"() -> (w3896:dbl)
                        n5463 = local write "Cible X"(w3898) -> ()
                        n5464 = local write "Cible Z"(w3896) -> ()
                        n5465 = local write "Cible Y"(w3897) -> ()
                        n5466 = local write "Calibration"(w3895) -> ()
                        n5467 = local write "Quit_Origine"(w3895) -> ()
                        n5468 = local write "RangeTable"(w3895) -> ()
                        n5469 = local write "Alacible"(w3895) -> ()
                        n5470 = local write "Origine"(w3895) -> ()
                        n5471 = local write "Centre"(w3895) -> ()
                      }
                    }
                  }
                }
              }
              event "StopTel": Value Change {
                # "Boucle de \nsurveillance du \nbouton STOP"
                n5472 = event-data() -> ("NewVal"=w3906:bool)  [unwired: 1 in, 4 out]
                n5473 = control-ref of="TERMINAL"() -> (w3904:refnum<vi>)
                n5474 = control-ref of="Indicateur d'état"() -> (w3905:refnum<vi>)
                n5475 = call "TERMINAL.vi"("Indicateur Refnum"=w3905, "Terminal Refnum"=w3904, "Indicateur d'état"="Appui du bouton \"STOP TÉL\"") -> ()
                n5476 = case shown="True" w3906 {
                  frame False {
                  }
                  frame True {
                    n5477 = flat-sequence {
                      tunnel: [w3932] -> w3907
                      frame #0 {
                        w3909 = FALSE ("Blinking")
                        w3911 = 0
                        w3912 = 0
                        w3913 = FALSE
                        n5478 = local read "Focus slew"() -> (w3908:bool)
                        n5479 = property on="GO" class="Bool (strict)"("Disabled"=w3912) -> ()  [unwired: 2 in, 2 out]
                        n5480 = property on="Zénith" class="Bool (strict)"("Disabled"=w3912) -> ()  [unwired: 2 in, 2 out]
                        n5481 = property on="Range" class="Bool (strict)"("Disabled"=w3912) -> ()  [unwired: 2 in, 2 out]
                        n5482 = property on="Écran" class="Bool (strict)"("Disabled"=w3912) -> ()  [unwired: 2 in, 2 out]
                        n5483 = property on="ModifRotation" class="Bool (strict)"("Disabled"=w3912) -> ()  [unwired: 2 in, 2 out]
                        n5484 = property on="ModifDome" class="Bool (strict)"("Disabled"=w3912) -> ()  [unwired: 2 in, 2 out]
                        n5485 = property on="StopTel" class="Bool (strict)"("Disabled"=w3912) -> ()  [unwired: 2 in, 2 out]
                        n5486 = case shown="True" w3908 {
                          frame False {
                          }
                          frame True {
                            "Annulation du foyer" <- TRUE
                          }
                        }
                        n5487 = local write "From library"(FALSE ("Déplacement usager")) -> ()
                        n5488 = property on="Offset OK" class="Bool (strict)"("Disabled"=w3911) -> ()  [unwired: 2 in, 2 out]
                        n5489 = property on="Coupole-Tél" class="Bool (strict)"("Disabled"=w3911) -> ()  [unwired: 2 in, 2 out]
                        n5490 = property on="ModCoor" class="Bool (strict)"("Disabled"=w3911) -> ()  [unwired: 2 in, 2 out]
                        n5491 = property on="ModifFoyer" class="Bool (strict)"("Disabled"=w3911) -> ()  [unwired: 2 in, 2 out]
                        n5492 = property on="Synctel" class="Bool (strict)"("Disabled"=w3911) -> ()  [unwired: 2 in, 2 out]
                        n5493 = local write "StopTel"(FALSE ("Raise Flag ?")) -> ()
                        n5494 = local write "Zénith"(w3913) -> ()
                        n5495 = local write "Écran"(w3913) -> ()
                        n5496 = local write "Range"(w3913) -> ()
